vi "getValFromVariant_enum.vi"(8 "error in (no error)":errorcluster, 10 "name":string, 11 "variant":variant) -> (0 "error out":errorcluster, 3 "value":string)   [LabVIEW 2018]
doc: "Get the value from variant (enum)."
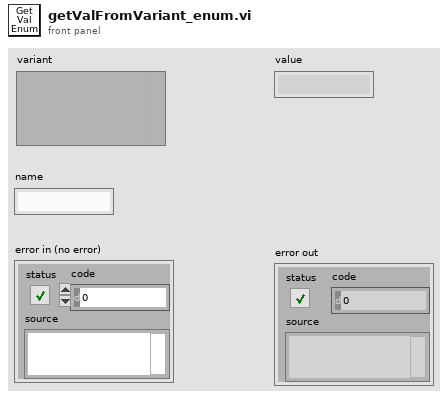
[diagram p1: front panel]
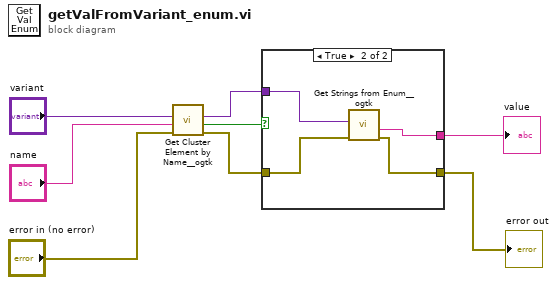
[diagram p0: block diagram]
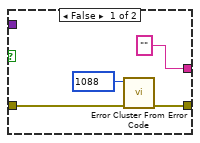
[diagram p2: hidden frame]
diagram:
  n1 = call <userlib>:"Get Cluster Element by Name__ogtk.vi"("error in (no error)"="error in (no error)", "Element Name"="name", "Cluster"="variant") -> ("error out"=w4:errorcluster, "found?"=w5:bool, "VElement"=w1:variant)  [unwired: 6 in]
  n2 = case shown="True" w5 {
    tunnel: w1 -> [_ w16]
    tunnel: w4 -> [w11 w15]
    tunnel: [w12 w14] -> w3
    tunnel: ["" ("data string") w13] -> w2
    frame False {
      n3 = call <vilib>:"Error Cluster From Error Code.vi"("error in (no error)"=w11, "error code (0)"=1088) -> ("error out"=w12:errorcluster)  [unwired: 7 in]
    }
    frame True {
      n4 = call <userlib>:"Get Strings from Enum__ogtk.vi"("error in (no error)"=w15, "Enum"=w16) -> ("error out"=w14:errorcluster, "String Value"=w13:string)  [unwired: 6 in, 2 out]
    }
  }
  "error out" <- w3
  "value" <- w2
